vi "Send Igor Command_MFP3D_Lucy.vi"(0 "Command":string="td_ReadValue(\"difference%laser\")", 3 "Expected output Format":string="%f") -> (7 "results":string="0.058594", 8 "History":string="%fprintf 0, \"%f\",td_ReadValue(\"difference%laser\")\r", 10 "error out":errorcluster)   [LabVIEW 2019]
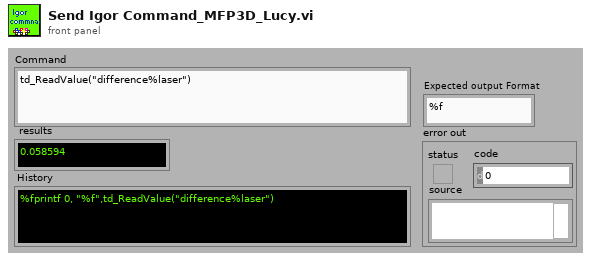
[diagram p1: front panel]
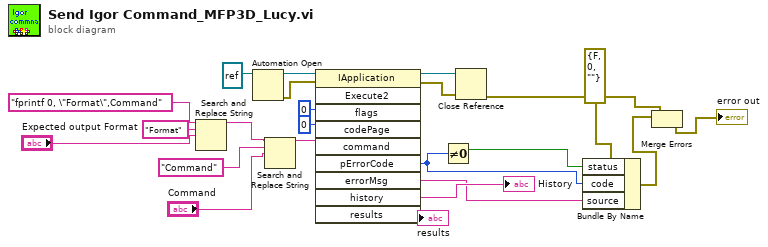
[diagram p0: block diagram]
diagram:
  n1 = Search and Replace String(input string="fprintf 0, \"Format\",Command" ("command"), search string="Format", replace string="Expected output Format") -> (result string=w12:string)  [unwired: 1 in, 7 out]
  n2 = Automation Open(Automation Refnum=refnum<k7> refnum ("IgorPro.IApplication")) -> (Automation Refnum=w23:refnum<k7>, error out=w22:errorcluster)  [unwired: 1 in, 2 out]
  n3 = Search and Replace String(input string=w12, search string="Command", replace string="Command") -> (result string=w9:string)  [unwired: 1 in, 7 out]
  n4 = invoke class="IApplication" method="Execute2"(reference=w23, error in=w22, "flags"=0, "codePage"=0, "command"=w9) -> (reference out=w21:refnum<k7>, error out=w20:errorcluster, "pErrorCode"=w4:i32, "errorMsg"=w3:string, "history"=→"History":string, "results"=→"results":string)  [unwired: 5 in, 4 out]
  n5 = Not Equal To 0?(x=w4) -> (x != 0?=w5:bool)
  n6 = Close Reference(reference=w21, error in (no error)=w20) -> (error out=w1:errorcluster)
  n7 = Bundle By Name(cluster=errorcluster {"status"=FALSE, "code"=0, "source"=""} ("error out 2"), "status"=w5, "code"=w4, "source"=w3) -> (w2:errorcluster)
  n8 = Merge Errors(w1, w2) -> (→"error out":errorcluster)
